vi "Read Attributes.vi"(11 "Abstract Message Template in":refnum<class "AAAA Msg.lvclass">) -> (2 "Payload":cluster{})   [LabVIEW 2016, in "AAAA Msg.lvclass"]
uses:
  AAAA Msg.lvclass
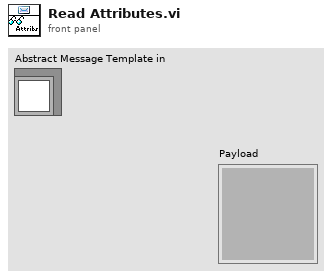
[diagram p1: front panel]
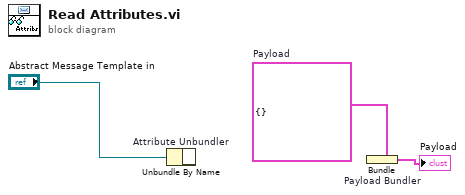
[diagram p0: block diagram]
diagram:
  w1 = cluster{} {}  # Payload
  n1 = Unbundle By Name "Attribute Unbundler"("Abstract Message Template in") -> ()  [unwired: 1 out]
  n2 = Bundle "Payload Bundler"(cluster=w1) -> (→"Payload":cluster{"Boolean":void})  [unwired: 1 in]
